vi "Manual Build.vi"(8 "Path to project":path, 9 "Path to repository":path, 10 "Package Version":string="2024.11.5.6", 11 "Product Name":string) -> (0 "Error Out":errorcluster)   [LabVIEW 2019, in "Build.lvlib"]
doc: "Use to build an (1) application (exe), (2) installer, and finally (3) a single 7z self-extracting installer file.\n\n<b>Product Name</b> is used in user dialog during product installation\n<b>Version</b> uses semantic versioning (Major.Minor.BugFix.Build)\n<b>Path to repository</b> points to the root directory of your repository; used to configure output build location\n<b>Path to project</b> points to the project containing build specifications"
uses:
  Build.lvlib
  PostBuildSupport/PostBuildSupport.lvclass
  <vilib>/MakerHub/Toolbox/LMH-Toolbox.lvlib
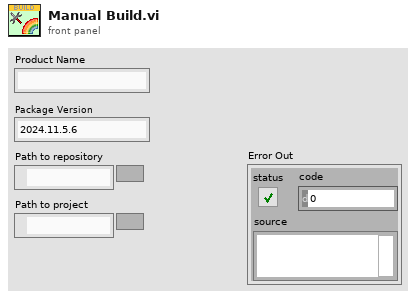
[diagram p1: front panel]
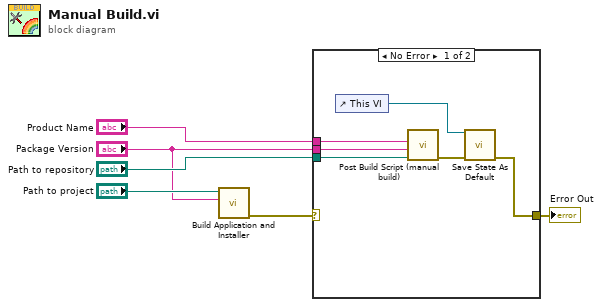
[diagram p0: block diagram]
diagram:
  n1 = call "Build Application and Installer.vi"("Package Version"="Package Version", "Path to project"="Path to project") -> ("error out"=w6:errorcluster)  [unwired: 9 in]
  n2 = case shown="No Error" w6 {
    selector: w6 -> [_ w13]
    tunnel: "Path to repository" -> [w10 _]
    tunnel: "Product Name" -> [w9 _]
    tunnel: "Package Version" -> [w8 _]
    tunnel: [w7 w13] -> w5
    frame No Error {
      n3 = control-ref of="This VI"() -> (w11:refnum<vi>)
      n4 = call "Post Build Script (manual build).vi"("Package Source Folder"=w10, "Package Version"=w8, "Product Name"=w9) -> ("error out"=w12:errorcluster)  [unwired: 8 in]
      n5 = call <vilib>:"Save State As Default.vi"("Error In"=w12, "Target VI"=w11) -> ("Error Out"=w7:errorcluster)  [unwired: 8 in, 1 out]
    }
    frame Error {
    }
  }
  "Error Out" <- w5
